vi "Test My Cloneable Module API.vi"() -> ()   [LabVIEW 2019]
doc: "My Module API Tester.\n_____\nBased on Delacor QMH Project Template 4.2.1.64."
uses:
  My Cloneable Module.lvlib
panel:
  in  "wait for reply":bool=TRUE
  in  "Run as Singleton?":bool
  in  "Show Block Diagram":bool
  in  "Refresh Modules":bool
  in  "X":dbl=1.0
  out "Reply Payload":dbl
  out "Active Modules":string[](array[string])
  in  "Stop Module":bool
  in  "Select Module":i32(ring)=-1 caption="Select Module\nTo send Request to" items=["All"=-1, "4140002"=4140002]
  in  "Run New Module":bool
  out "Do Something Count":i32
  in  "Test Do Something Else and Wait for Reply":bool
  in  "Hide Module Panel":bool
  in  "Show Module Panel":bool
  in  "Test Do Something Else":bool
  in  "Test Do Something":bool
  out "Status":string
  # "This VI tests the API for the Module."
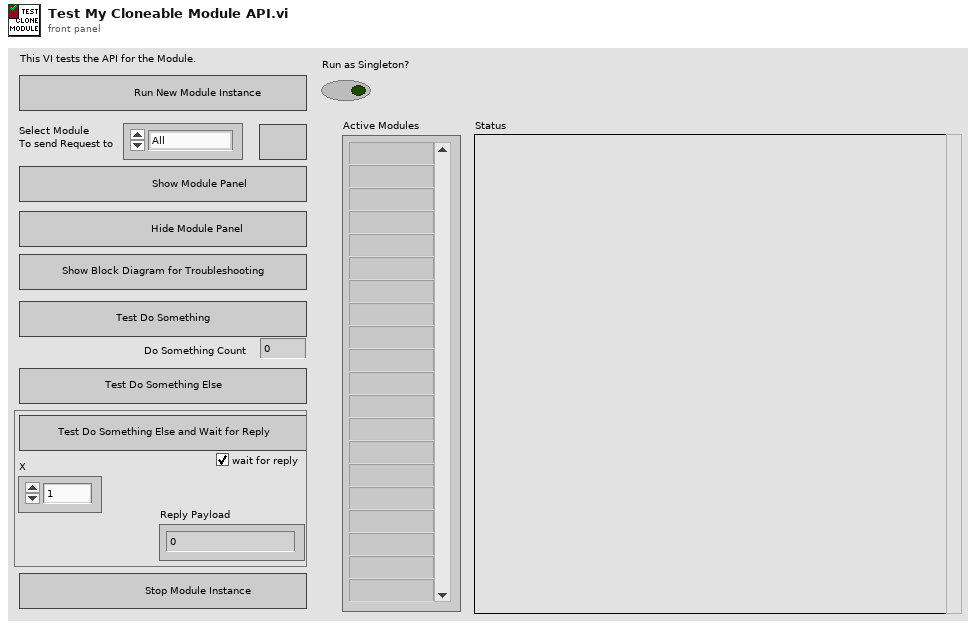
[diagram p1: front panel]
types:
  T1 = typedef "My Cloneable Module.lvlib/Broadcast Events--cluster.ctl" = cluster{"Module Did Init":refnum<user-event>, "Status Updated":refnum<user-event>, "Error Reported":refnum<user-event>, "Did Something":refnum<user-event>, "Module Did Stop":refnum<user-event>, "Update Module Execution Status":refnum<user-event>}
  T2 = typedef "My Cloneable Module.lvlib/Do Something Else and Wait (Reply Payload)--cluster.ctl" = cluster{"Value":dbl, "error":errorcluster}
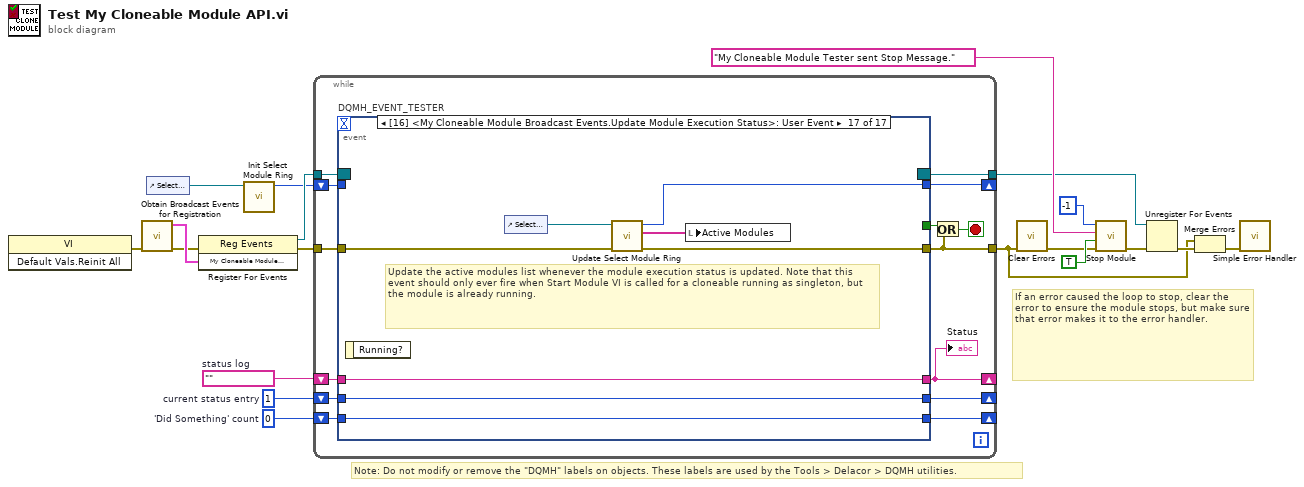
[diagram p0: block diagram]
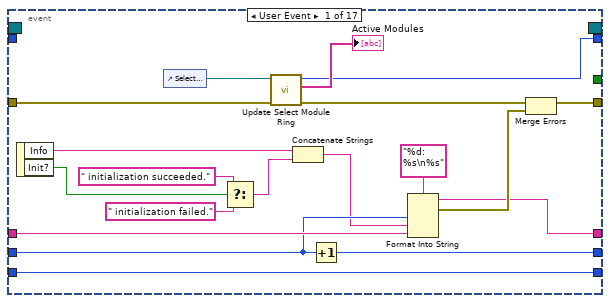
[diagram p2: hidden frame]
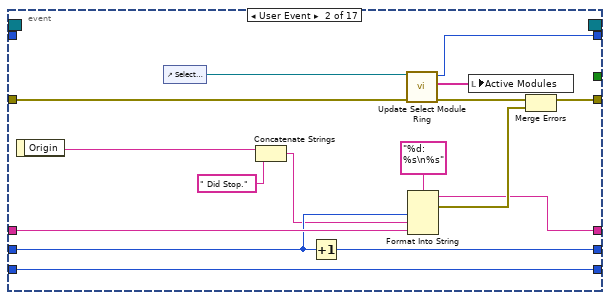
[diagram p3: hidden frame]
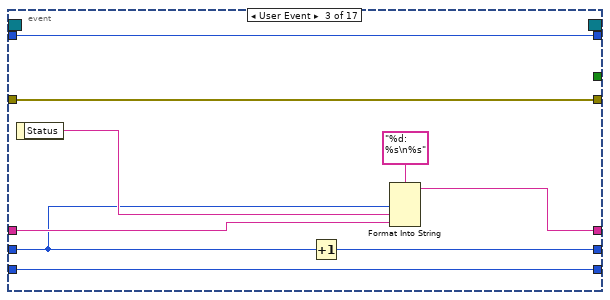
[diagram p4: hidden frame]
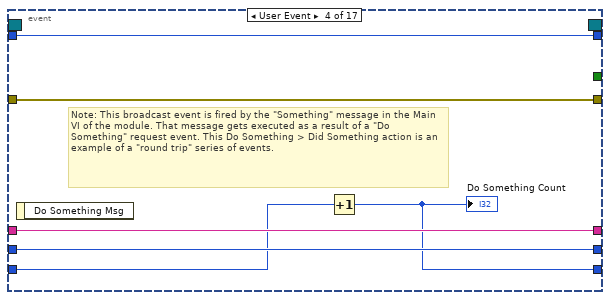
[diagram p5: hidden frame]
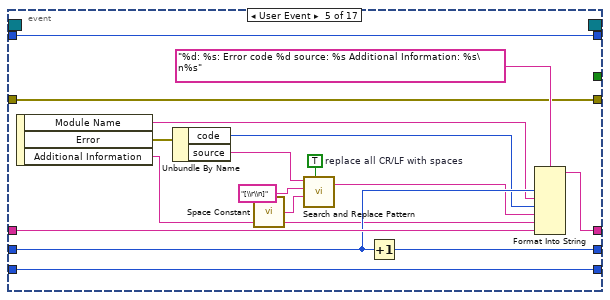
[diagram p6: hidden frame]
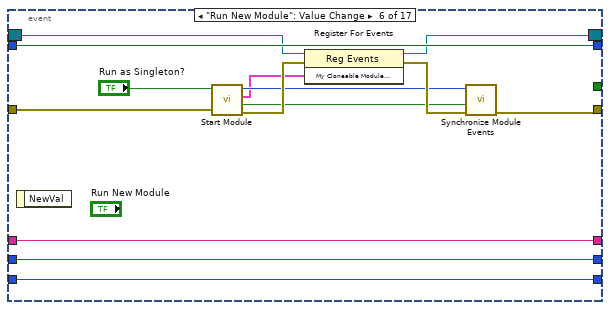
[diagram p7: hidden frame]
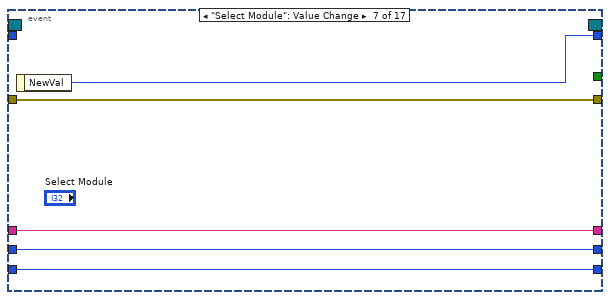
[diagram p8: hidden frame]
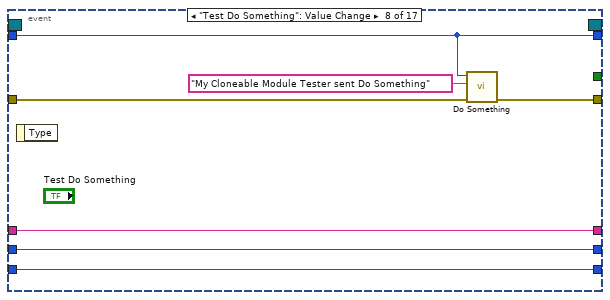
[diagram p9: hidden frame]
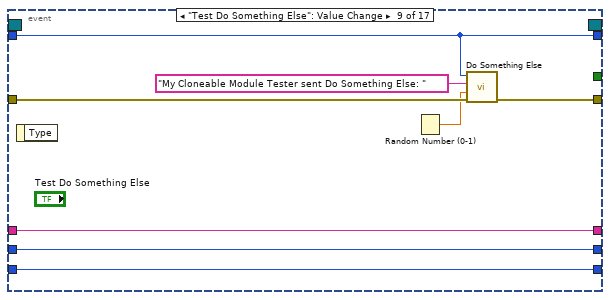
[diagram p10: hidden frame]
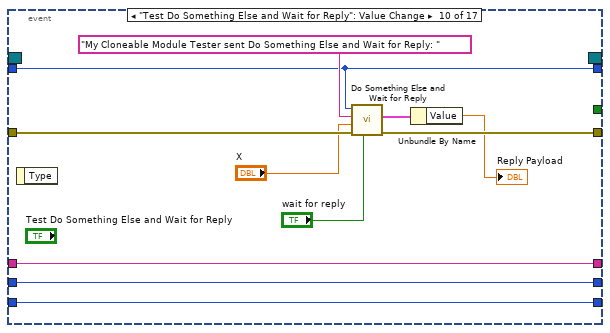
[diagram p11: hidden frame]
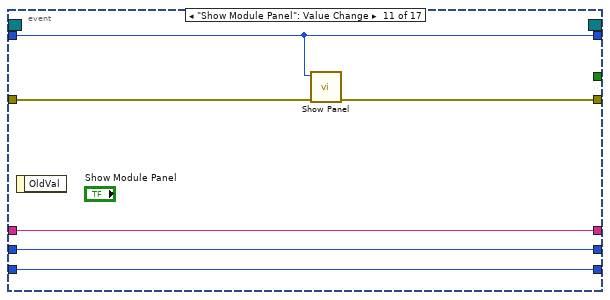
[diagram p12: hidden frame]
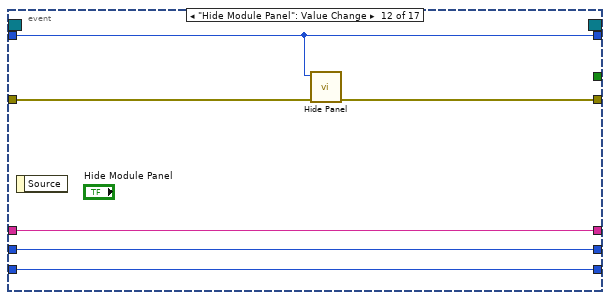
[diagram p13: hidden frame]
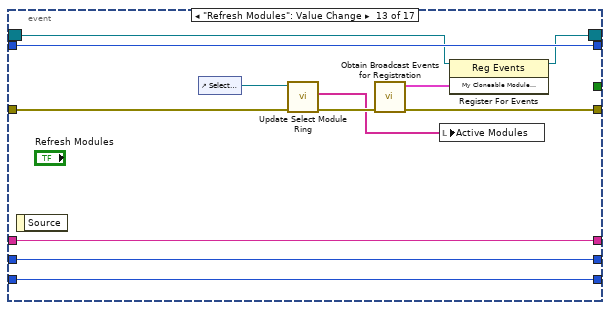
[diagram p14: hidden frame]
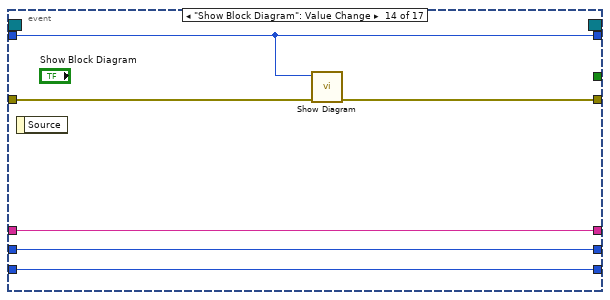
[diagram p15: hidden frame]
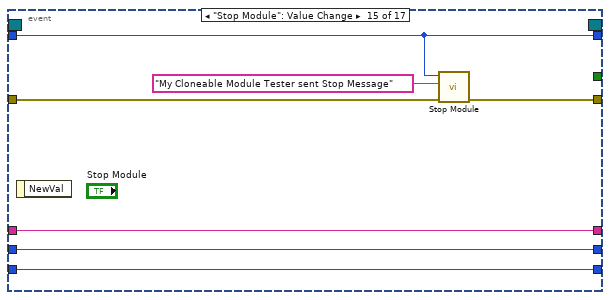
[diagram p16: hidden frame]
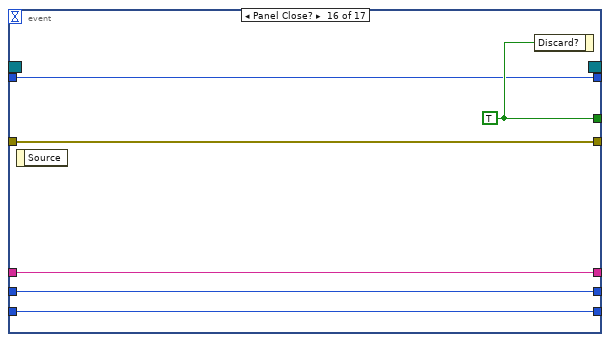
[diagram p17: hidden frame]
diagram:
  w14 = 0  # 'Did Something' count
  w15 = 1  # current status entry
  w16 = ""  # status log
  # "If an error caused the loop to stop, clear the error to ensure the module stops, but make sure that error makes it to the error handler."
  # "Note: Do not modify or remove the \"DQMH\" labels on objects. These labels are used by the Tools > Delacor > DQMH utilities."
  n1 = invoke class="VI" method="Default Vals.Reinit All"() -> (error out=w2:errorcluster)  [unwired: 3 in, 2 out]
  n2 = call "Obtain Broadcast Events for Registration.vi"("error in (no error)"=w2) -> ("error out"=w1:errorcluster, "My Cloneable Module Broadcast Events"=w11:T1)  [unwired: 9 in]
  n3 = control-ref of="Select Module"() -> (w12:refnum<vi>)
  n4 = register-events(error in=w1, w11) -> (reference out=w19:refnum<event-registration>, error out=w10:errorcluster)  [unwired: 1 in]
  n5 = call "Init Select Module Ring.vi"("Select Module Ring Ref"=w12) -> ("Value for All Modules"=w13:i32)  [unwired: 8 in, 2 out]
  n6 = while {
    tunnel: w19 -> [w33]
    tunnel: [w20] -> w3
    tunnel: w10 -> [w31]
    shift-right: [w27] -> _
    shift-left: w16 -> [w29]
    shift-right: [w28] -> _
    shift-left: w15 -> [w30]
    shift-right: [w25] -> _
    shift-left: w14 -> [w26]
    shift-right: [w22] -> _
    shift-left: w13 -> [w23]
    tunnel: [w21] -> w7
    stop <- w24 stop-if-true
    n7 = event "DQMH_EVENT_TESTER" shown="[16] <My Cloneable Module Broadcast Events.Update Module Execution Status>: User Event" {
      selector: w33 -> [_ _ _ _ _ w107 _ _ _ _ _ _ w163 _ _ _ _]
      dyn-events: [_ _ _ _ _ w106 _ _ _ _ _ _ w162 _ _ _ _] -> w21
      timeout: _ -> [_ _ _ _ _ _ _ _ _ _ _ _ _ _ _ _ _]
      tunnel: [_ _ _ _ _ _ _ _ _ _ _ _ _ _ _ w188 _] -> w32
      tunnel: [w41 w59 w77 w83 w89 w105 w119 w125 w133 w145 w150 w156 w159 w171 w177 w187 w191] -> w20
      tunnel: w31 -> [w43 w61 w77 w83 w89 w108 w119 w126 w134 w137 w151 w157 w164 w175 w178 w187 w192]
      tunnel: w30 -> [w49 w65 w69 w81 w95 w111 w117 w122 w129 w142 w148 w154 w168 w173 w181 w185 w195]
      tunnel: w29 -> [w50 w66 w73 w82 w97 w112 w118 w123 w130 w143 w149 w155 w169 w174 w182 w186 w196]
      tunnel: [w47 w63 w74 w82 w92 w112 w118 w123 w130 w143 w149 w155 w169 w174 w182 w186 w196] -> w27
      tunnel: [w48 w64 w76 w81 w98 w111 w117 w122 w129 w142 w148 w154 w168 w173 w181 w185 w195] -> w28
      tunnel: w26 -> [w44 w62 w72 w80 w100 w110 w116 w121 w128 w141 w147 w153 w167 w172 w180 w184 w194]
      tunnel: [w44 w62 w72 w79 w100 w110 w116 w121 w128 w141 w147 w153 w167 w172 w180 w184 w194] -> w25
      tunnel: w23 -> [_ _ w70 w78 w99 w109 _ w120 w127 w140 w146 w152 w166 w170 w179 w183 _]
      tunnel: [w38 w56 w70 w78 w99 w109 w115 w120 w127 w140 w146 w152 w166 w170 w179 w183 w190] -> w22
      event User Event {
        n8 = event-data() -> ("Info"=w46:string, "Init?"=w35:bool)  [unwired: 1 in]
        n9 = control-ref of="Select Module"() -> (w40:refnum<vi>)
        n10 = Select(t=" initialization succeeded.", s=w35, f=" initialization failed.") -> (s? t:f=w34:string)
        n11 = call "Update Select Module Ring.vi"("error in (no error)"=w43, "Select Module Ring Ref"=w40) -> ("error out"=w42:errorcluster, "Active Modules (Array)"=→"Active Modules":string[], "New Module Ring Value"=w38:i32)  [unwired: 7 in]
        n12 = Concatenate Strings(w46, w34) -> (w45:string)
        n13 = Increment(x=w49) -> (x+1=w48:i32)
        n14 = Format Into String(format string="%d: %s\n%s", w49, w45, w50) -> (resulting string=w47:string, error out=w52:errorcluster)  [unwired: 2 in]
        n15 = Merge Errors(w42, w52) -> (w41:errorcluster)
      }
      event User Event {
        n16 = event-data() -> ("Origin"=w54:string)  [unwired: 1 in]
        n17 = control-ref of="Select Module"() -> (w58:refnum<vi>)
        n18 = Concatenate Strings(w54, " Did Stop.") -> (w53:string)
        n19 = Increment(x=w65) -> (x+1=w64:i32)
        n20 = call "Update Select Module Ring.vi"("error in (no error)"=w61, "Select Module Ring Ref"=w58) -> ("error out"=w60:errorcluster, "Active Modules (Array)"=w57:string[], "New Module Ring Value"=w56:i32)  [unwired: 7 in]
        n21 = Format Into String(format string="%d: %s\n%s", w65, w53, w66) -> (resulting string=w63:string, error out=w68:errorcluster)  [unwired: 2 in]
        n22 = local write "Active Modules"(w57) -> ()
        n23 = Merge Errors(w60, w68) -> (w59:errorcluster)
      }
      event User Event {
        n24 = event-data() -> ("Status"=w71:string)  [unwired: 1 in]
        n25 = Increment(x=w69) -> (x+1=w76:i32)
        n26 = Format Into String(format string="%d: %s\n%s", w69, w71, w73) -> (resulting string=w74:string)  [unwired: 2 in, 1 out]
      }
      event User Event {
        # "Note: This broadcast event is fired by the \"Something\" message in the Main VI of the module. That message gets executed as a result of a \"Do Something\" request event. This Do Something > Did Something action is an example of a \"round trip\" series of events."
        n27 = event-data() -> ()  [unwired: 1 in, 1 out]
        n28 = Increment(x=w80) -> (x+1=w79:i32)
        "Do Something Count" <- w79
      }
      event User Event {
        w93 = TRUE  # replace all CR/LF with spaces
        n29 = event-data() -> ("Module Name"=w87:string, "Error"=w86:errorcluster, "Additional Information"=w84:string)  [unwired: 1 in]
        n30 = Unbundle By Name(w86) -> ("code"=w88:i32, "source"=w90:string)
        n31 = call <vilib>:"Space Constant.vi"() -> ("String"=w94:string)
        n32 = call <vilib>:"Search and Replace Pattern.vi"("string"=w90, "regular expression (\"\")"="[\\r\\n]" ("regular expression (\"\")"), "replace string (\"\")"=w94, "replace all? (F)"=w93) -> ("result string"=w91:string)  [unwired: 1 in, 1 out]
        n33 = Increment(x=w95) -> (x+1=w98:i32)
        n34 = Format Into String(format string="%d: %s: Error code %d source: %s Additional Information: %s\n%s", w95, w87, w88, w91, w84, w97) -> (resulting string=w92:string)  [unwired: 2 in, 1 out]
      }
      event "Run New Module": Value Change {
        n35 = event-data() -> ()  [unwired: 1 in, 1 out]
        n36 = call "Start Module.vi"("error in (no error)"=w108, "Run as Singleton? (F)"="Run as Singleton?") -> ("error out"=w113:errorcluster, "Wait for Event Sync?"=w103:bool, "My Cloneable Module Broadcast Events"=w102:T1, "Module ID"=w104:i32)  [unwired: 6 in]
        n37 = register-events(reference=w107, error in=w113, w102) -> (reference out=w106:refnum<event-registration>, error out=w114:errorcluster)
        n38 = call "Synchronize Module Events.vi"("error in (no error)"=w114, "Wait for Event Sync?"=w103, "Module ID"=w104) -> ("error out"=w105:errorcluster)  [unwired: 7 in, 1 out]
      }
      event "Select Module": Value Change {
        n39 = event-data() -> ("NewVal"=w115:i32)  [unwired: 1 in]
      }
      event "Test Do Something": Value Change {
        n40 = event-data() -> ()  [unwired: 1 in, 1 out]
        n41 = call "Do Something.vi"("error in (no error)"=w126, "Do Something Message"="My Cloneable Module Tester sent Do Something", "Module ID"=w120) -> ("error out"=w125:errorcluster)  [unwired: 8 in]
      }
      event "Test Do Something Else": Value Change {
        n42 = event-data() -> ()  [unwired: 1 in, 1 out]
        n43 = Random Number (0-1)() -> (number: 0 to 1=w131:dbl)
        n44 = call "Do Something Else.vi"("error in (no error)"=w134, "X"=w131, "Do Something else Message"="My Cloneable Module Tester sent Do Something Else: " ("Do Something Message"), "Module ID"=w127) -> ("error out"=w133:errorcluster)  [unwired: 7 in]
      }
      event "Test Do Something Else and Wait for Reply": Value Change {
        n45 = event-data() -> ()  [unwired: 1 in, 1 out]
        n46 = call "Do Something Else and Wait for Reply.vi"("wait for reply (T)"="wait for reply", "error in (no error)"=w137, "X"="X", "Do Something Else Message"="My Cloneable Module Tester sent Do Something Else and Wait for Reply: " ("Do Something Message"), "Module ID"=w140) -> ("error out"=w145:errorcluster, "Reply Payload"=w139:T2)  [unwired: 4 in, 1 out]
        n47 = Unbundle By Name(w139) -> ("Value"=→"Reply Payload":dbl)
      }
      event "Show Module Panel": Value Change {
        n48 = event-data() -> ()  [unwired: 1 in, 1 out]
        n49 = call "Show Panel.vi"("error in (no error)"=w151, "Module ID"=w146) -> ("error out"=w150:errorcluster)  [unwired: 9 in]
      }
      event "Hide Module Panel": Value Change {
        n50 = event-data() -> ()  [unwired: 1 in, 1 out]
        n51 = call "Hide Panel.vi"("error in (no error)"=w157, "Module ID"=w152) -> ("error out"=w156:errorcluster)  [unwired: 9 in]
      }
      event "Refresh Modules": Value Change {
        n52 = event-data() -> ()  [unwired: 1 in, 1 out]
        n53 = control-ref of="Select Module"() -> (w165:refnum<vi>)
        n54 = call "Update Select Module Ring.vi"("error in (no error)"=w164, "Select Module Ring Ref"=w165) -> ("error out"=w160:errorcluster, "Active Modules (Array)"=w158:string[])  [unwired: 7 in, 1 out]
        n55 = call "Obtain Broadcast Events for Registration.vi"("error in (no error)"=w160) -> ("error out"=w159:errorcluster, "My Cloneable Module Broadcast Events"=w161:T1)  [unwired: 9 in]
        n56 = local write "Active Modules"(w158) -> ()
        n57 = register-events(reference=w163, w161) -> (reference out=w162:refnum<event-registration>)  [unwired: 1 in, 1 out]
      }
      event "Show Block Diagram": Value Change {
        n58 = event-data() -> ()  [unwired: 1 in, 1 out]
        n59 = call "Show Diagram.vi"("error in (no error)"=w175, "Module ID"=w170) -> ("error out"=w171:errorcluster)  [unwired: 9 in]
      }
      event "Stop Module": Value Change {
        n60 = event-data() -> ()  [unwired: 1 in, 1 out]
        n61 = call "Stop Module.vi"("error in (no error)"=w178, "Origin"="My Cloneable Module Tester sent Stop Message", "Module ID"=w179) -> ("error out"=w177:errorcluster)  [unwired: 8 in]
      }
      event Panel Close? {
        w188 = TRUE ("Discard?")
        n62 = event-data() -> ()  [unwired: 1 in, 1 out]
        n63 = event-data("Discard?"=w188) -> ()  [unwired: 1 in, 1 out]
      }
      event User Event {
        # "Update the active modules list whenever the module execution status is updated. Note that this event should only ever fire when Start Module VI is called for a cloneable running as singleton, but the module is already running."
        n64 = event-data() -> ()  [unwired: 1 in, 1 out]
        n65 = control-ref of="Select Module"() -> (w193:refnum<vi>)
        n66 = call "Update Select Module Ring.vi"("error in (no error)"=w192, "Select Module Ring Ref"=w193) -> ("error out"=w191:errorcluster, "Active Modules (Array)"=w189:string[], "New Module Ring Value"=w190:i32)  [unwired: 7 in]
        n67 = local write "Active Modules"(w189) -> ()
      }
    }
    "Status" <- w27
    n68 = Or(x=w32, y=w20) -> (x .or. y?=w24:bool)
  }
  n69 = call <vilib>:"Clear Errors.vi"("error in (no error)"=w3) -> ("error out"=w5:errorcluster)  [unwired: 5 in, 1 out]
  n70 = call "Stop Module.vi"("error in (no error)"=w5, "Wait for Module to stop? (F)"=TRUE ("Wait for Module to stop?"), "Origin"="My Cloneable Module Tester sent Stop Message.", "Module ID"=-1 ("Stop all")) -> ("error out"=w17:errorcluster)  [unwired: 7 in]
  n71 = Unregister For Events(event registration refnum=w7, error in=w17) -> (error out=w18:errorcluster)
  n72 = Merge Errors(w3, w18) -> (w4:errorcluster)
  n73 = call <vilib>:"Simple Error Handler.vi"("error in (no error)"=w4) -> ()  [unwired: 4 in, 5 out]
